vi "Set vacuum.vi"(8 "error in (no error)":errorcluster, 10 "Vacuum?":bool, 11 "Pressure Control in":refnum<class "Pressure Control.lvclass">) -> (0 "error out":errorcluster, 3 "Pressure Control out":refnum<class "Pressure Control.lvclass">)   [LabVIEW 2011, in "Pressure Control.lvclass"]
uses:
  Pressure Control.lvclass
  Pressure Control.lvclass/Pressure Control.ctl
  TTL/TTL.lvclass
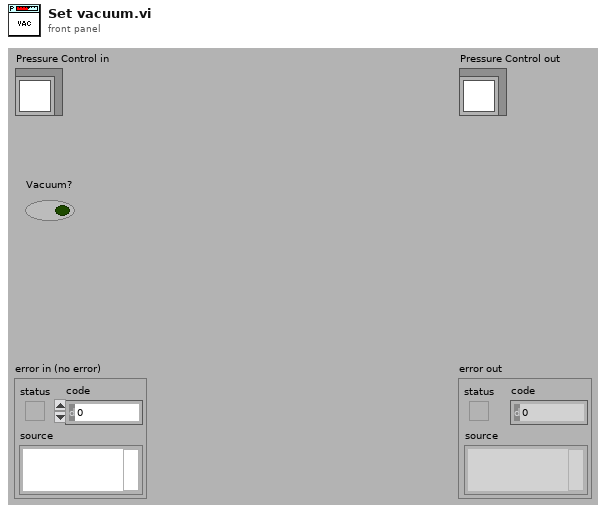
[diagram p1: front panel]
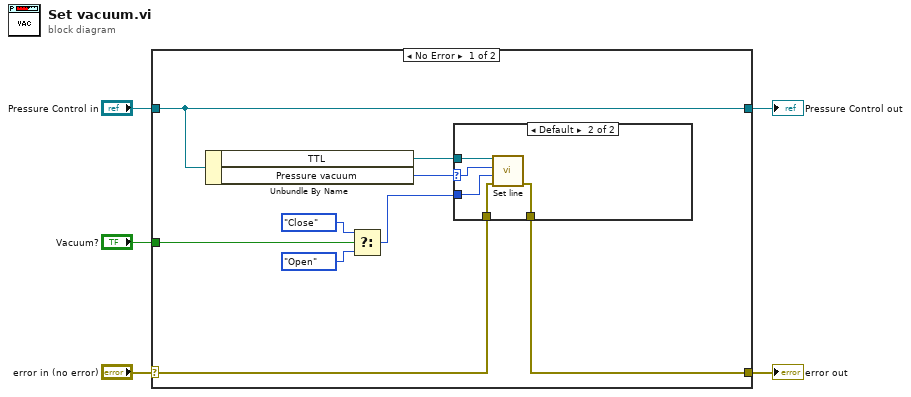
[diagram p0: block diagram]
diagram:
  n1 = case shown="No Error" "error in (no error)" {
    selector: "error in (no error)" -> [w12 w22]
    tunnel: [w11 w22] -> w4
    tunnel: [w14 w21] -> w2
    tunnel: "Pressure Control in" -> [w14 w21]
    tunnel: "Vacuum?" -> [w9 _]
    frame No Error {
      n2 = Unbundle By Name(w14) -> ("TTL"=w13:refnum<class "TTL.lvclass">, "Pressure vacuum"=w10:i32)
      n3 = Select(t=enum16{"Open", "Close", "Toggle"}."Close" ("Action"), s=w9, f=enum16{"Open", "Close", "Toggle"}."Open" ("Action")) -> (s? t:f=w6:enum16{"Open", "Close", "Toggle"})
      n4 = case shown="Default" w10 {
        selector: w10 -> [_ w17]
        tunnel: w13 -> [_ w20]
        tunnel: w12 -> [w15 w19]
        tunnel: [w15 w18] -> w11
        tunnel: w6 -> [_ w16]
        frame -1 {
          # "No \"vacuum\" line was defined\nin the hardware config"
        }
        frame Default {
          n5 = call "Set line.vi"("error in (no error)"=w19, "Action"=w16, "Line number"=w17, "TTL in"=w20) -> ("error out"=w18:errorcluster)  [unwired: 6 in, 1 out]
        }
      }
    }
    frame Error {
    }
  }
  "error out" <- w4
  "Pressure Control out" <- w2
